vi "tm431_regionofinterest.vi"() -> ()   [LabVIEW 2011]
panel:
  out "Software FPS":dbl
  out "Camera FPS":dbl
  out "Image":u16[][](graph)
  out "SVW":i32
  out "SHW":i32
  out "SVO":i32
  out "SHO":i32
  in  "V Width":i32 min=4 max=2048 step=4
  in  "V Offset":i32 min=0 max=0 step=4
  in  "H Width":i32 min=4 max=2048 step=4
  in  "H Offset":i32 min=0 max=0 step=4
  in  "Binning":i32(ring)=1 items=["1x1"=1, "2x2"=2, "4x4"=4]
  out "error out":errorcluster
  in  "stop":bool
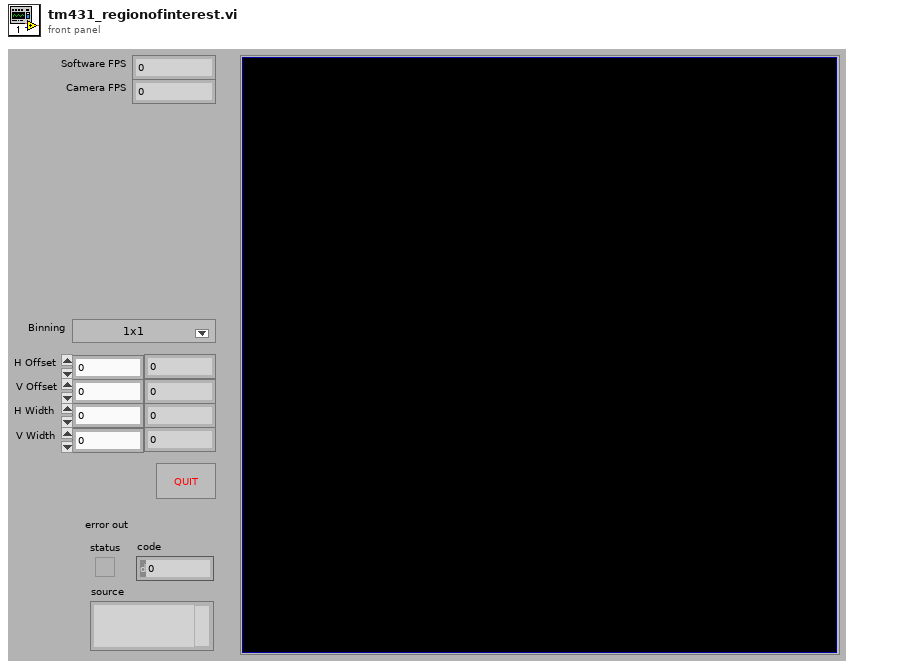
[diagram p1: front panel]
types:
  T1 = typedef "LVMinMaxIncTypeDef.ctl" = cluster{"Minimum":dbl, "Maximum":dbl, "Increment":dbl}
  T2 = cluster{"H Offset":cluster{"Value":i32, "Limits":T1}, "V Offset":cluster{"Value":i32, "Limits":T1}, "H Size":cluster{"Value":i32, "Limits":T1}, "V Size":cluster{"Value":i32, "Limits":T1}}
  T3 = cluster{"H Offset":i32, "V Offset":i32, "H Width":i32, "V Width":i32}
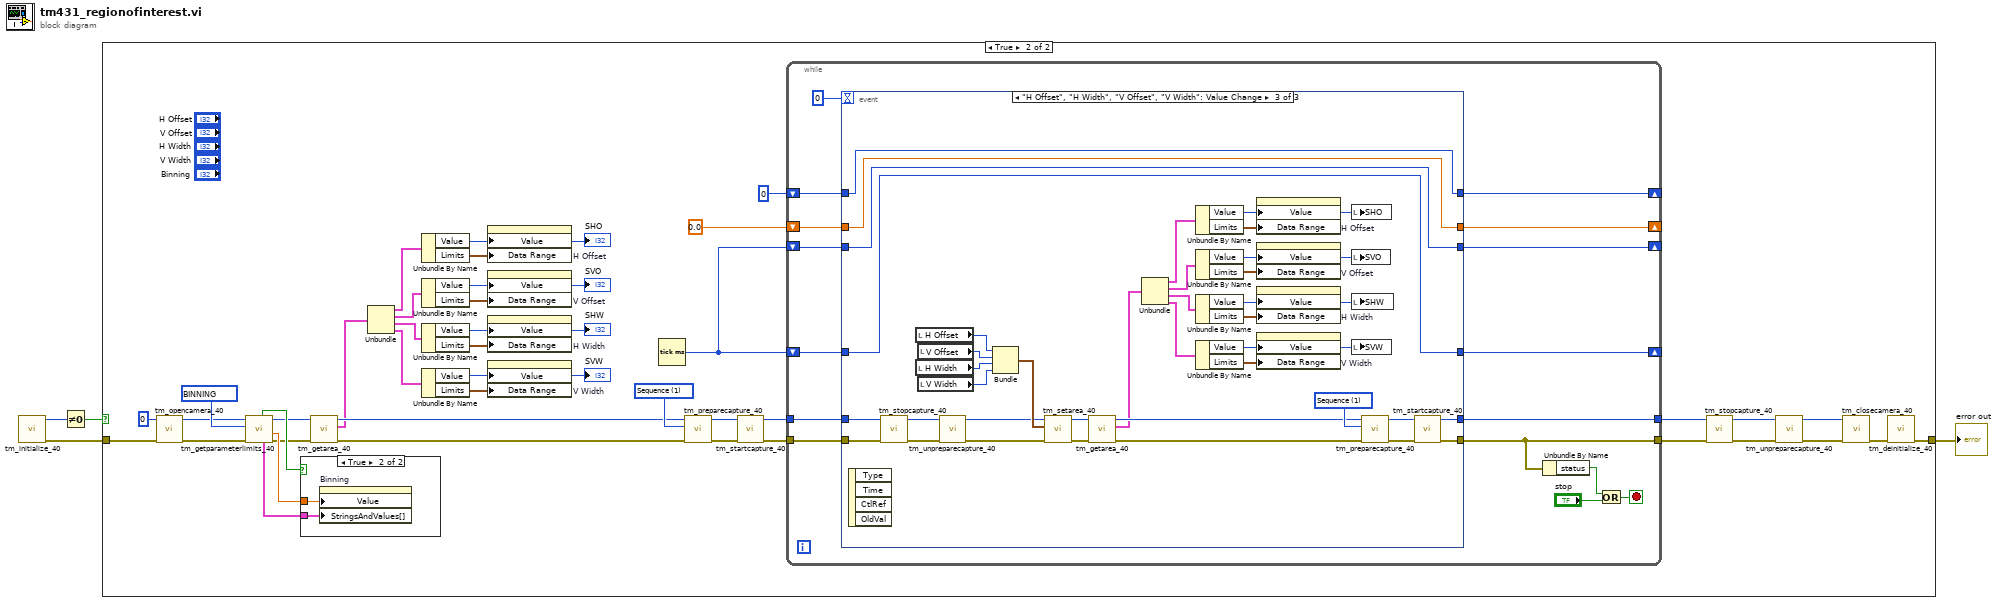
[diagram p0: block diagram]
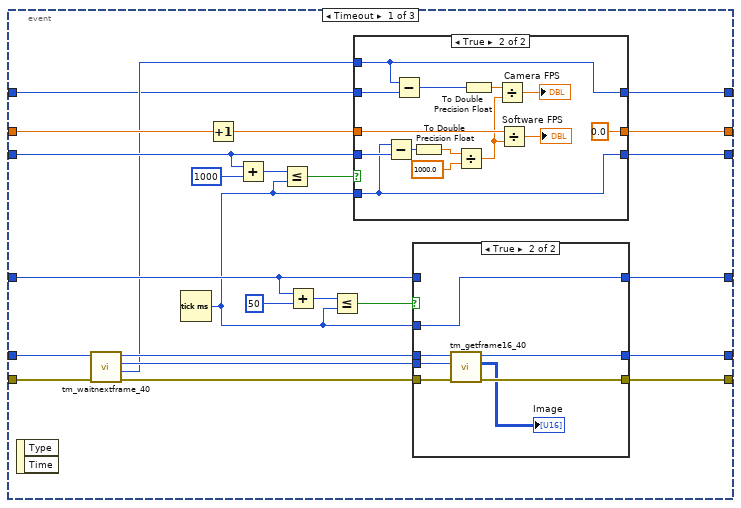
[diagram p4: hidden frame]
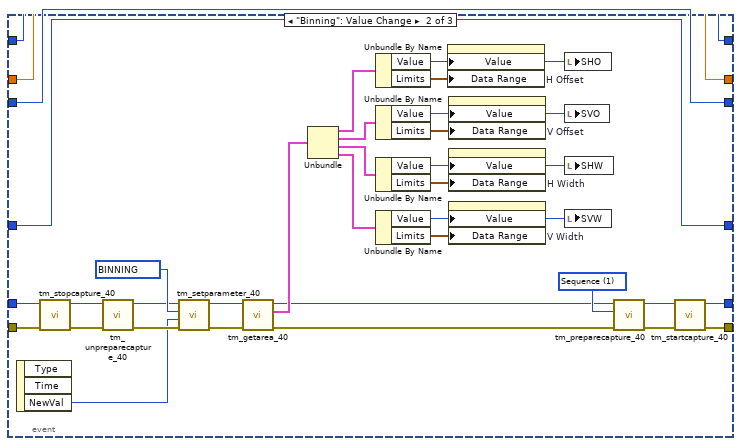
[diagram p7: hidden frame]
diagram:
  n1 = call <userlib>:"tm_initialize_40.vi"() -> ("error out"=w2:errorcluster, "Number Of Cameras"=w1:u32)  [unwired: 8 in, 2 out]
  n2 = Not Equal To 0?(x=w1) -> (x != 0?=w4:bool)
  n3 = case shown="True" w4 {
    tunnel: [w5 w43] -> w3
    tunnel: w2 -> [w5 w46]
    frame False {
    }
    frame True {
      w25 = u32 4215968 items=["BINNING"=4215968, "BITS PER CHANNEL"=4342976, "ACTIVE VIEW INDEX"=4343136, "CCD MODE"=4212384, "SENSOR MODE"=4212128, "READOUT MODE"=4211872, "EXPOSURE TIME"=2049184, "CONTRAST GAIN"=3163312, "CONTRAST OFFSET"=3163328, "LIGHT MODE"=2114720, "SENSITIVITY"=2114992, "WHITE BALANCE"=3163568, "PHOTON IMAGING MODE"=2115200, "HIGH DYNAMIC RANGE MODE"=3163360, "TRIGGER SOURCE"=1066144, "TRIGGER ACTIVE"=1066160, "TRIGGER MODE"=1066400, "TRIGGER POLARITY"=1066416, "TRIGGER GLOBAL EXPOSURE"=2049680, "FIRST TRIGGER BEHAVIOR"=2049696, "TRIGGER TIMES"=1066448, "OUTPUT TRIGGER POLARITY"=1852592, "OUTPUT TRIGGER DELAY"=1852624, "OUTPUT TRIGGER PERIOD"=1852640, "TEMPERATURE"=2115232, "TEMPERATURE TARGET"=2115264, "SENSOR COOLER FAN"=2115296, "MECHANICAL SHUTTER"=2115488, "BACK FOCUS POSITION"=8422304, "FRAMEBUNDLE MODE"=4346784, "FRAMEBUNDLE NUMBER"=4346800, "LINEBUNDLE HEIGHT"=4212192, "TRIGGER CONNECTOR"=1066432, "IMAGE PIXEL TYPE"=4343296, "OUTPUT TRIGGER KIND"=1852656, "READOUT DIRECTION"=4211904, "CHANNEL SYNC"=1852352] ("Parameter")
      w41 = 1 items=["Snap", "Sequence"] ("Capture mode")
      n4 = call <userlib>:"tm_opencamera_40.vi"("error in (no error)"=w46, "Camera Index"=u32 0) -> ("error out"=w20:errorcluster, "Handle out"=w19:u32)  [unwired: 7 in, 1 out]
      n5 = call <userlib>:"tm_getparameterlimits_40.vi"("error in (no error)"=w20, "Parameter"=w25, "Handle in"=w19) -> ("error out"=w24:errorcluster, "default"=w27:dbl, "Handle out"=w23:u32, "Value Names"=w26:cluster{"Name":string, "Value":dbl}[], "Writable"=w28:bool)  [unwired: 2 in, 2 out]
      n6 = case shown="True" w28 {
        tunnel: w26 -> [_ w48]
        tunnel: w27 -> [_ w47]
        frame False {
        }
        frame True {
          n7 = property on="Binning" class="Ring (strict)"("Value"=w47, "StringsAndValues[]"=w48) -> ()  [unwired: 2 in, 2 out]
        }
      }
      n8 = call <userlib>:"tm_getarea_40.vi"("error in (no error)"=w24, "Handle in"=w23) -> ("error out"=w22:errorcluster, "Sub Region"=w14:T2, "Handle out"=w21:u32)  [unwired: 7 in]
      n9 = Unbundle(w14) -> ("H Offset"=w18:cluster{"Value":i32, "Limits":T1}, "V Offset"=w17:cluster{"Value":i32, "Limits":T1}, "H Size"=w16:cluster{"Value":i32, "Limits":T1}, "V Size"=w15:cluster{"Value":i32, "Limits":T1})
      n10 = Unbundle By Name(w18) -> ("Value"=w13:i32, "Limits"=w11:T1)
      "SHO" <- w13
      n11 = Unbundle By Name(w17) -> ("Value"=w10:i32, "Limits"=w9:T1)
      "SVO" <- w10
      n12 = Unbundle By Name(w16) -> ("Value"=w8:i32, "Limits"=w7:T1)
      "SHW" <- w8
      n13 = Unbundle By Name(w15) -> ("Value"=w12:i32, "Limits"=w6:T1)
      "SVW" <- w12
      n14 = property on="H Offset" class="DigNum (strict)"("Value"=w13, "Data Range"=w11) -> ()  [unwired: 2 in, 2 out]
      n15 = property on="V Offset" class="DigNum (strict)"("Value"=w10, "Data Range"=w9) -> ()  [unwired: 2 in, 2 out]
      n16 = property on="H Width" class="DigNum (strict)"("Value"=w8, "Data Range"=w7) -> ()  [unwired: 2 in, 2 out]
      n17 = property on="V Width" class="DigNum (strict)"("Value"=w12, "Data Range"=w6) -> ()  [unwired: 2 in, 2 out]
      n18 = Tick Count (ms)() -> (millisecond timer value=w36:u32)
      n19 = call <userlib>:"tm_preparecapture_40.vi"("error in (no error)"=w22, "Capture mode"=w41, "Handle in"=w21) -> ("error out"=w39:errorcluster, "Handle out"=w40:u32)  [unwired: 5 in, 2 out]
      n20 = call <userlib>:"tm_startcapture_40.vi"("error in (no error)"=w39, "Handle in"=w40) -> ("error out"=w38:errorcluster, "Handle out"=w37:u32)  [unwired: 8 in]
      n21 = while {
        tunnel: w38 -> [w55]
        tunnel: [w53] -> w35
        tunnel: [w52] -> w34
        shift-right: [w60] -> _
        shift-left: w36 -> [w58]
        shift-right: [w61] -> _
        shift-left: 0.0 -> [w59]
        shift-right: [w54] -> _
        shift-left: w36 -> [w57]
        tunnel: w37 -> [w56]
        shift-right: [w49] -> _
        shift-left: 0 -> [w50]
        stop <- w62 stop-if-true
        n22 = event shown="[2] \"H Offset\", \"H Width\", \"V Offset\", \"V Width\": Value Change" {
          selector: _ -> [_ _ _]
          dyn-events: _ -> [_ _ _]
          timeout: 0 -> [_ _ _]
          tunnel: [w70 w142 w179] -> w61
          tunnel: [w69 w143 w180] -> w60
          tunnel: w59 -> [w78 w142 w179]
          tunnel: w58 -> [w72 w143 w180]
          tunnel: w57 -> [w79 w149 w186]
          tunnel: w56 -> [w81 w141 w173]
          tunnel: w55 -> [w80 w140 w172]
          tunnel: [w77 w149 w186] -> w54
          tunnel: [w76 w144 w181] -> w53
          tunnel: [w75 w145 w182] -> w52
          tunnel: w50 -> [w67 w137 w167]
          tunnel: [w66 w137 w167] -> w49
          event Timeout {
            n23 = event-data() -> ()  [unwired: 1 in, 2 out]
            n24 = call <userlib>:"tm_waitnextframe_40.vi"("error in (no error)"=w80, "Handle in"=w81) -> ("error out"=w83:errorcluster, "Frame Count"=w68:i32, "Frame Index"=w82:i32, "Handle out"=w84:u32)  [unwired: 6 in]
            n25 = Tick Count (ms)() -> (millisecond timer value=w74:u32)
            n26 = Increment(x=w78) -> (x+1=w71:dbl)
            n27 = Add(x=w72, y=u32 1000) -> (x+y=w88:u32)
            n28 = Less Or Equal?(x=w88, y=w74) -> (x <= y?=w73:bool)
            n29 = Add(x=w79, y=u32 50) -> (x+y=w86:u32)
            n30 = Less Or Equal?(x=w86, y=w74) -> (x <= y?=w65:bool)
            n31 = case shown="True" w73 {
              tunnel: w72 -> [w91 w100]
              tunnel: [w91 w97] -> w69
              tunnel: w71 -> [w90 w103]
              tunnel: w74 -> [_ w97]
              tunnel: [w90 0.0] -> w70
              tunnel: w68 -> [_ w92]
              tunnel: w67 -> [w89 w95]
              tunnel: [w89 w92] -> w66
              frame False {
              }
              frame True {
                n32 = Subtract(x=w97, y=w100) -> (x-y=w99:u32)
                n33 = Subtract(x=w92, y=w95) -> (x-y=w93:i32)
                n34 = To Double Precision Float(number=w99) -> (double precision float=w105:dbl)
                n35 = Divide(x=w105, y=1000.0) -> (x/y=w96:dbl)
                n36 = To Double Precision Float(number=w93) -> (double precision float=w94:dbl)
                n37 = Divide(x=w94, y=w96) -> (x/y=→"Camera FPS":dbl)
                n38 = Divide(x=w103, y=w96) -> (x/y=→"Software FPS":dbl)
              }
            }
            n39 = case shown="True" w65 {
              tunnel: w79 -> [w108 _]
              tunnel: w74 -> [_ w115]
              tunnel: [w108 w115] -> w77
              tunnel: w84 -> [w107 w114]
              tunnel: w83 -> [w106 w113]
              tunnel: [w107 w112] -> w76
              tunnel: [w106 w111] -> w75
              tunnel: w82 -> [_ w109]
              frame False {
              }
              frame True {
                n40 = call <userlib>:"tm_getframe16_40.vi"("error in (no error)"=w113, "Frame Index"=w109, "Handle in"=w114) -> ("error out"=w111:errorcluster, "Data"=→"Image":u16[][], "Handle out"=w112:u32)  [unwired: 5 in, 1 out]
              }
            }
          }
          event "Binning": Value Change {
            w135 = u32 4215968 items=["BINNING"=4215968, "BITS PER CHANNEL"=2, "ACTIVE VIEW INDEX"=3, "CCD MODE"=4, "SENSOR MODE"=5, "READOUT MODE"=6, "EXPOSURE TIME"=7, "CONTRAST GAIN"=8, "CONTRAST OFFSET"=9, "LIGHT MODE"=10, "SENSITIVITY"=11, "WHITE BALANCE"=12, "PHOTON IMAGING MODE"=13, "HIGH DYNAMIC RANGE MODE"=14, "TRIGGER SOURCE"=15, "TRIGGER ACTIVE"=16, "TRIGGER MODE"=17, "TRIGGER POLARITY"=18, "TRIGGER GLOBAL EXPOSURE"=19, "FIRST TRIGGER BEHAVIOR"=20, "TRIGGER TIMES"=21, "OUTPUT TRIGGER POLARITY"=22, "OUTPUT TRIGGER DELAY"=23, "OUTPUT TRIGGER PERIOD"=24, "TEMPERATURE"=25, "TEMPERATURE TARGET"=26, "SENSOR COOLER FAN"=27, "MECHANICAL SHUTTER"=28, "BACK FOCUS POSITION"=29, "FRAMEBUNDLE MODE"=30, "FRAMEBUNDLE NUMBER"=31, "LINEBUNDLE HEIGHT"=32, "TRIGGER CONNECTOR"=33, "IMAGE PIXEL TYPE"=34, "OUTPUT TRIGGER KIND"=35, "READOUT DIRECTION"=36, "CHANNEL SYNC"=37] ("Parameter")
            w148 = 1 items=["Snap", "Sequence"] ("Capture mode")
            n41 = event-data() -> ("NewVal"=w133:i32)  [unwired: 1 in, 2 out]
            n42 = call <userlib>:"tm_stopcapture_40.vi"("error in (no error)"=w140, "Handle in"=w141) -> ("error out"=w138:errorcluster, "Handle out"=w139:u32)  [unwired: 8 in]
            n43 = call <userlib>:"tm_unpreparecapture_40.vi"("error in (no error)"=w138, "Handle in"=w139) -> ("error out"=w136:errorcluster, "Handle out"=w134:u32)  [unwired: 8 in]
            n44 = call <userlib>:"tm_setparameter_40.vi"("error in (no error)"=w136, "Value in"=w133, "Parameter"=w135, "Handle in"=w134) -> ("error out"=w130:errorcluster, "Handle out"=w131:u32)  [unwired: 6 in]
            n45 = call <userlib>:"tm_getarea_40.vi"("error in (no error)"=w130, "Handle in"=w131) -> ("error out"=w128:errorcluster, "Sub Region"=w132:T2, "Handle out"=w129:u32)  [unwired: 7 in]
            n46 = Unbundle(w132) -> ("H Offset"=w127:cluster{"Value":i32, "Limits":T1}, "V Offset"=w118:cluster{"Value":i32, "Limits":T1}, "H Size"=w116:cluster{"Value":i32, "Limits":T1}, "V Size"=w117:cluster{"Value":i32, "Limits":T1})
            n47 = Unbundle By Name(w127) -> ("Value"=w126:i32, "Limits"=w125:T1)
            n48 = Unbundle By Name(w118) -> ("Value"=w122:i32, "Limits"=w121:T1)
            n49 = Unbundle By Name(w116) -> ("Value"=w120:i32, "Limits"=w119:T1)
            n50 = Unbundle By Name(w117) -> ("Value"=w124:i32, "Limits"=w123:T1)
            n51 = property on="H Offset" class="DigNum (strict)"("Value"=w126, "Data Range"=w125) -> ()  [unwired: 2 in, 2 out]
            n52 = property on="V Offset" class="DigNum (strict)"("Value"=w122, "Data Range"=w121) -> ()  [unwired: 2 in, 2 out]
            n53 = property on="H Width" class="DigNum (strict)"("Value"=w120, "Data Range"=w119) -> ()  [unwired: 2 in, 2 out]
            n54 = property on="V Width" class="DigNum (strict)"("Value"=w124, "Data Range"=w123) -> ()  [unwired: 2 in, 2 out]
            n55 = local write "SHO"(w126) -> ()
            n56 = local write "SVO"(w122) -> ()
            n57 = local write "SHW"(w120) -> ()
            n58 = local write "SVW"(w124) -> ()
            n59 = call <userlib>:"tm_preparecapture_40.vi"("error in (no error)"=w128, "Capture mode"=w148, "Handle in"=w129) -> ("error out"=w146:errorcluster, "Handle out"=w147:u32)  [unwired: 5 in, 2 out]
            n60 = call <userlib>:"tm_startcapture_40.vi"("error in (no error)"=w146, "Handle in"=w147) -> ("error out"=w145:errorcluster, "Handle out"=w144:u32)  [unwired: 8 in]
          }
          event "H Offset", "H Width", "V Offset", "V Width": Value Change {
            w185 = 1 items=["Snap", "Sequence"] ("Capture mode")
            n61 = event-data() -> ()  [unwired: 1 in, 4 out]
            n62 = call <userlib>:"tm_stopcapture_40.vi"("error in (no error)"=w172, "Handle in"=w173) -> ("error out"=w170:errorcluster, "Handle out"=w171:u32)  [unwired: 8 in]
            n63 = local read "H Offset"() -> (w176:i32)
            n64 = local read "H Width"() -> (w177:i32)
            n65 = local read "V Offset"() -> (w178:i32)
            n66 = local read "V Width"() -> (w175:i32)
            n67 = call <userlib>:"tm_unpreparecapture_40.vi"("error in (no error)"=w170, "Handle in"=w171) -> ("error out"=w168:errorcluster, "Handle out"=w169:u32)  [unwired: 8 in]
            n68 = Bundle("H Offset"=w176, "V Offset"=w178, "H Width"=w177, "V Width"=w175) -> (w174:T3)  [unwired: 1 in]
            n69 = call <userlib>:"tm_setarea_40.vi"("error in (no error)"=w168, "Sub Region"=w174, "Handle in"=w169) -> ("error out"=w165:errorcluster, "Handle out"=w166:u32)  [unwired: 7 in]
            n70 = call <userlib>:"tm_getarea_40.vi"("error in (no error)"=w165, "Handle in"=w166) -> ("error out"=w163:errorcluster, "Sub Region"=w162:T2, "Handle out"=w164:u32)  [unwired: 7 in]
            n71 = Unbundle(w162) -> ("H Offset"=w161:cluster{"Value":i32, "Limits":T1}, "V Offset"=w152:cluster{"Value":i32, "Limits":T1}, "H Size"=w151:cluster{"Value":i32, "Limits":T1}, "V Size"=w150:cluster{"Value":i32, "Limits":T1})
            n72 = Unbundle By Name(w161) -> ("Value"=w160:i32, "Limits"=w159:T1)
            n73 = Unbundle By Name(w152) -> ("Value"=w158:i32, "Limits"=w157:T1)
            n74 = Unbundle By Name(w151) -> ("Value"=w156:i32, "Limits"=w155:T1)
            n75 = Unbundle By Name(w150) -> ("Value"=w154:i32, "Limits"=w153:T1)
            n76 = property on="H Offset" class="DigNum (strict)"("Value"=w160, "Data Range"=w159) -> ()  [unwired: 2 in, 2 out]
            n77 = property on="V Offset" class="DigNum (strict)"("Value"=w158, "Data Range"=w157) -> ()  [unwired: 2 in, 2 out]
            n78 = property on="H Width" class="DigNum (strict)"("Value"=w156, "Data Range"=w155) -> ()  [unwired: 2 in, 2 out]
            n79 = property on="V Width" class="DigNum (strict)"("Value"=w154, "Data Range"=w153) -> ()  [unwired: 2 in, 2 out]
            n80 = local write "SHO"(w160) -> ()
            n81 = local write "SVO"(w158) -> ()
            n82 = local write "SHW"(w156) -> ()
            n83 = local write "SVW"(w154) -> ()
            n84 = call <userlib>:"tm_preparecapture_40.vi"("error in (no error)"=w163, "Capture mode"=w185, "Handle in"=w164) -> ("error out"=w183:errorcluster, "Handle out"=w184:u32)  [unwired: 5 in, 2 out]
            n85 = call <userlib>:"tm_startcapture_40.vi"("error in (no error)"=w183, "Handle in"=w184) -> ("error out"=w182:errorcluster, "Handle out"=w181:u32)  [unwired: 8 in]
          }
        }
        n86 = Unbundle By Name(w52) -> ("status"=w63:bool)
        n87 = Or(x=w63, y="stop") -> (x .or. y?=w62:bool)
      }
      n88 = call <userlib>:"tm_stopcapture_40.vi"("error in (no error)"=w34, "Handle in"=w35) -> ("error out"=w31:errorcluster, "Handle out"=w32:u32)  [unwired: 8 in]
      n89 = call <userlib>:"tm_unpreparecapture_40.vi"("error in (no error)"=w31, "Handle in"=w32) -> ("error out"=w30:errorcluster, "Handle out"=w33:u32)  [unwired: 8 in]
      n90 = call <userlib>:"tm_closecamera_40.vi"("error in (no error)"=w30, "Handle in"=w33) -> ("error out"=w44:errorcluster)  [unwired: 9 in]
      n91 = call <userlib>:"tm_deinitialize_40.vi"("error in (no error)"=w44) -> ("error out"=w43:errorcluster)  [unwired: 10 in]
    }
  }
  "error out" <- w3
